vi "Disabled.vi"(7 "Robot Mode":T2, 10 "Match Info":T1={"Autonomous Elapsed Seconds"=0.0, "TeleOp Elapsed Seconds"=0.0, "Disabled Elapsed Seconds"=0.0, "Visited Autonomous"=FALSE, "Visited TeleOp"=FALSE, "Visited Disabled"=FALSE, "Autonomous Settings"={"Autonomous Style"=enum."Independent", "VI Refnum"=refnum}}, 11 "Call Context":T3) -> ()   [LabVIEW 2011]
doc: "This VI is called each time a disabled packet is received from the DS. It is often used to prepare for the next robot mode, to calibrate sensors, etc."
uses:
  <vilib>/Rock Robotics/WPI/DriverStation/WPI_DriverStationDerivedRobotMode.ctl
  <vilib>/Rock Robotics/WPI/DriverStation/WPI_DriverStationRobotMode.ctl
  <vilib>/Rock Robotics/WPI/DriverStation/WPI_DriverStationMatch Info.ctl
  Robot Global Data.vi
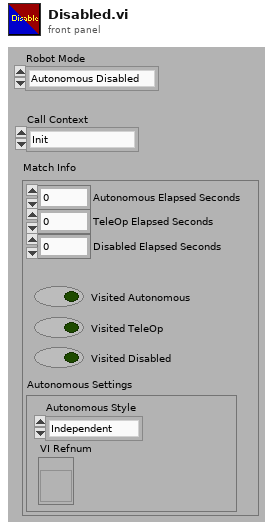
[diagram p1: front panel]
types:
  T1 = typedef "WPI_DriverStationMatch Info.ctl" = cluster{"Autonomous Elapsed Seconds":dbl, "TeleOp Elapsed Seconds":dbl, "Disabled Elapsed Seconds":dbl, "Visited Autonomous":bool, "Visited TeleOp":bool, "Visited Disabled":bool, "Autonomous Settings":cluster{"Autonomous Style":enum16{"Iterative", "Independent"}, "VI Refnum":refnum<vi>}}
  T2 = typedef "WPI_DriverStationRobotMode.ctl" = enum16{"Autonomous Disabled", "Autonomous Enabled", "Teleop Disabled", "Teleop Enabled", "Timeout", "Finish"}
  T3 = typedef "WPI_DriverStationDerivedRobotMode.ctl" = enum16{"Init", "Execute", "Stop"}
  T4 = typedef "WPI_JoystickDevRef.ctl" = cluster{"Device":T5}
  T5 = typedef "WPI_JoystickDeviceEnum.ctl" = enum16{"USB 1", "USB 2", "USB 3", "USB 4", "Kinect 1", "Kinect 2"}
  T6 = typedef "WPI_JoystickButtonState.ctl" = cluster{"Button 1":bool, "Button 2":bool, "Button 3":bool, "Button 4":bool, "Button 5":bool, "Button 6":bool, "Button 7":bool, "Button 8":bool, "Button 9":bool, "Button 10":bool, "Button 11":bool, "Button 12":bool}
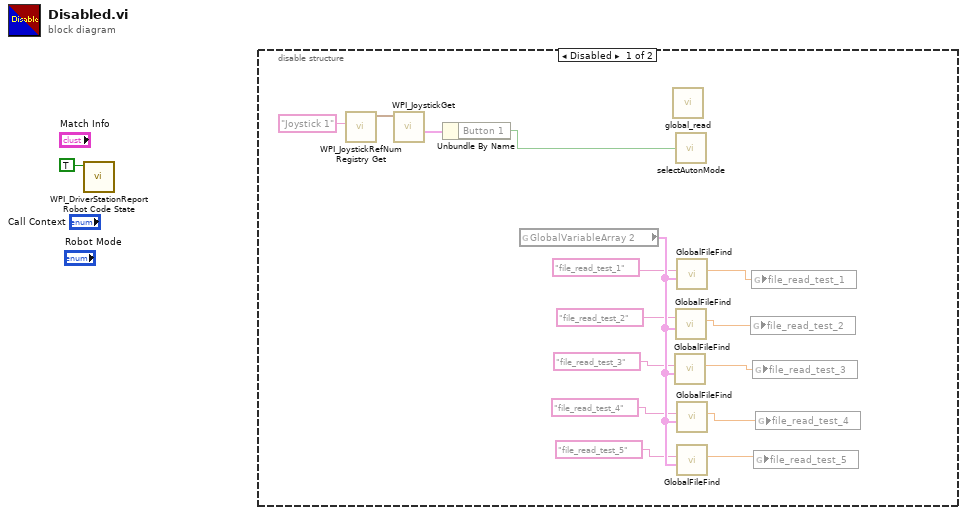
[diagram p0: block diagram]
diagram:
  n1 = call <vilib>:"WPI_DriverStationReport Robot Code State.vi"("Disabled"=TRUE ("Autonomous")) -> ()  [unwired: 10 in, 1 out]
  n2 = disable-structure shown="Disabled" {
    frame Disabled {
      n3 = call <vilib>:"WPI_JoystickRefNum Registry Get.vi"("refnum name"="Joystick 1") -> ("JoystickDevRef"=w15:T4)  [unwired: 9 in, 1 out]
      n4 = call <vilib>:"WPI_JoystickGet.vi"("JoystickDevRef"=w15) -> ("Buttons"=w14:T6)  [unwired: 4 in, 2 out]
      n5 = Unbundle By Name(w14) -> ("Button 1"=w13:bool)
      n6 = global read "Robot Global Data.vi" "GlobalVariableArray 2"() -> (w12:cluster{"name":string, "va;":dbl}[])
      n7 = call "global_read.vi"() -> ()  [unwired: 12 in]
      n8 = call "GlobalFileFind.vi"("GlobalVariableArray 2"=w12, "VariableNameLookup"="file_read_test_3") -> ("VariableValueOut"=w3:dbl)  [unwired: 9 in]
      n9 = call "selectAutonMode.vi"("Joystick"=w13) -> ()  [unwired: 1 in]
      n10 = call "GlobalFileFind.vi"("GlobalVariableArray 2"=w12, "VariableNameLookup"="file_read_test_2") -> ("VariableValueOut"=w2:dbl)  [unwired: 9 in]
      n11 = call "GlobalFileFind.vi"("GlobalVariableArray 2"=w12, "VariableNameLookup"="file_read_test_1") -> ("VariableValueOut"=w6:dbl)  [unwired: 9 in]
      n12 = call "GlobalFileFind.vi"("GlobalVariableArray 2"=w12, "VariableNameLookup"="file_read_test_4") -> ("VariableValueOut"=w4:dbl)  [unwired: 9 in]
      n13 = call "GlobalFileFind.vi"("GlobalVariableArray 2"=w12, "VariableNameLookup"="file_read_test_5") -> ("VariableValueOut"=w5:dbl)  [unwired: 9 in]
      n14 = global write "Robot Global Data.vi" "file_read_test_2"(w2) -> ()
      n15 = global write "Robot Global Data.vi" "file_read_test_1"(w6) -> ()
      n16 = global write "Robot Global Data.vi" "file_read_test_3"(w3) -> ()
      n17 = global write "Robot Global Data.vi" "file_read_test_5"(w5) -> ()
      n18 = global write "Robot Global Data.vi" "file_read_test_4"(w4) -> ()
    }
    frame Enabled {
    }
  }
